vi "Robot Global Data.vi"() -> ()   [LabVIEW 2017]
doc: "This global VI can contain as many global variables as you need. Place a control on the panel, give it a good name. To read or write to it from a VI, drag the icon to the diagram of that VI. You can also drag from the project. Click on the node to change which global you access. You shouldn't have multiple locations writing to a global or it will cause a race-condition."
uses:
  <vilib>/Rock Robotics/WPI/Camera/WPI_CameraImageSize.ctl
  <vilib>/Rock Robotics/WPI/DriverStation/WPI_DriverStationRobotMode2.ctl
  <vilib>/Rock Robotics/WPI/Solenoid/WPI_SolenoidValue.ctl
  <vilib>/Rock Robotics/WPI/DriverStation/WPI_DriverStationMatch Info.ctl
panel:
  in  "Angle at Start of Auto":dbl
  in  "Place From Null":bool
  in  "Auto Selector":string
  in  "Auto Arm Fast":bool
  in  "Lift Down Speed Fast":dbl=-0.9
  in  "Lift Down Fast":bool=TRUE
  in  "Auto Running":dbl=-1.0
  in  "Scale Position":string
  in  "Switch Position":string
  in  "Attempt 2 Cube":bool
  in  "Do Not Cross Field":bool
  in  "Focus Switch":bool
  in  "Have Cube?":bool
  in  "Arm Auto Min Speed":bool
  in  "Cube Sensor":dbl
  in  "Arm Encoder New Reading":dbl
  in  "Auto Scale Drive Forward Distance":dbl=300.0
  in  "Arm Encoder Offset":dbl
  in  "Climbing Override":bool
  in  "Encoders to use":u16(ring)=2 items=["Use Both Encoders", "Use Just Right Encoder", "Use Just Left Encoder"]
  in  "Rollover":dbl
  in  "Continuos Yaw":dbl
  in  "Lift Max Height":dbl=67.0
  out "Match Info":T1={"Autonomous Elapsed Seconds"=0.0, "TeleOp Elapsed Seconds"=0.0, "Disabled Elapsed Seconds"=0.0, "Visited Autonomous"=FALSE, "Visited TeleOp"=FALSE, "Visited Disabled"=FALSE, "Autonomous Settings"={"Autonomous Style"=enum."Independent", "VI Refnum"=refnum}}
  in  "Intake Speed Override":dbl
  in  "Intake Indicator":bool
  in  "Intake Pistons":T2
  in  "Arm Manual Speed":dbl
  in  "Arm Manual Control":bool=TRUE
  in  "LED Control Pattern":dbl=0.27
  in  "LEDs on Robot":bool
  in  "Lift Manual Control":bool
  in  "Lift Manual Speed":dbl
  in  "Intake Speed":dbl
  in  "Right Climber Piston":bool
  in  "Left Climber Piston":bool
  in  "Right Ski Piston":bool
  in  "Left Ski Piston":bool
  in  "Arm Back Limit Switch":bool
  in  "Arm Front Limit Switch":bool
  in  "Lift Encoder Stopped":bool
  in  "Lift Encoder Rate":dbl
  in  "Left Bottom Lift Limit Switch":bool
  in  "Right Bottom Lift Limit Switch":bool
  in  "Left Top Lift Limit Switch":bool
  in  "Right Top Lift Limit Switch":bool
  in  "Lift Encoder Distance":dbl
  in  "Skis on Robot":bool
  in  "Climber on Robot":bool
  in  "Drive on Robot":bool=TRUE
  in  "Intake on Robot":bool=TRUE
  in  "Lift on Robot":bool=TRUE
  in  "Arm on Robot":bool=TRUE
  in  "Practice Bot?":bool
  in  "Compressor Stop":bool
  in  "Lift Height to rase to (in)":dbl
  in  "Lift Max Speed to Raise at (%)":dbl=1.0
  in  "Arm Max Speed to Turn at":dbl
  in  "Arm Angle to Turn to":dbl=3000.0
  in  "Arm Encoder Reading":dbl
  in  "Limelight Pipeline":dbl
  in  "Limelight Cam Mode":dbl=1.0
  in  "Limelight Led Mode":dbl=1.0
  in  "Right Drive Encoder Stopped":bool
  in  "Right Drive Encoder Rate":dbl
  in  "Right Drive Encoder Distance":dbl
  in  "Left Drive Encoder Stopped":bool
  in  "Left Drive Encoder Rate":dbl
  in  "Left Drive Encoder Distance":dbl
  in  "Limelight Data":T3
  in  "Robot Drive Y":dbl
  in  "Robot Drive X":dbl
  in  "Fused Heading":dbl
  in  "Heading":dbl
  in  "Pitch":dbl
  in  "Roll":dbl
  in  "Yaw":dbl
  in  "image size":T4=enum."320x240"
  in  "Enable Vision":bool
  in  "Robot Mode":T5
  # "0 Both\n1 Right\n2 Left"
  # "Navx Data"
  # "Limelight Controls"
  # "Drive Encoders"
  # "Arm"
  # "Items on Robot"
  # "Intake"
  # "Skis"
  # "Climber"
  # "Pnuematics"
  # "Robot Drive Setpoints"
  # "Driver Camera Settings"
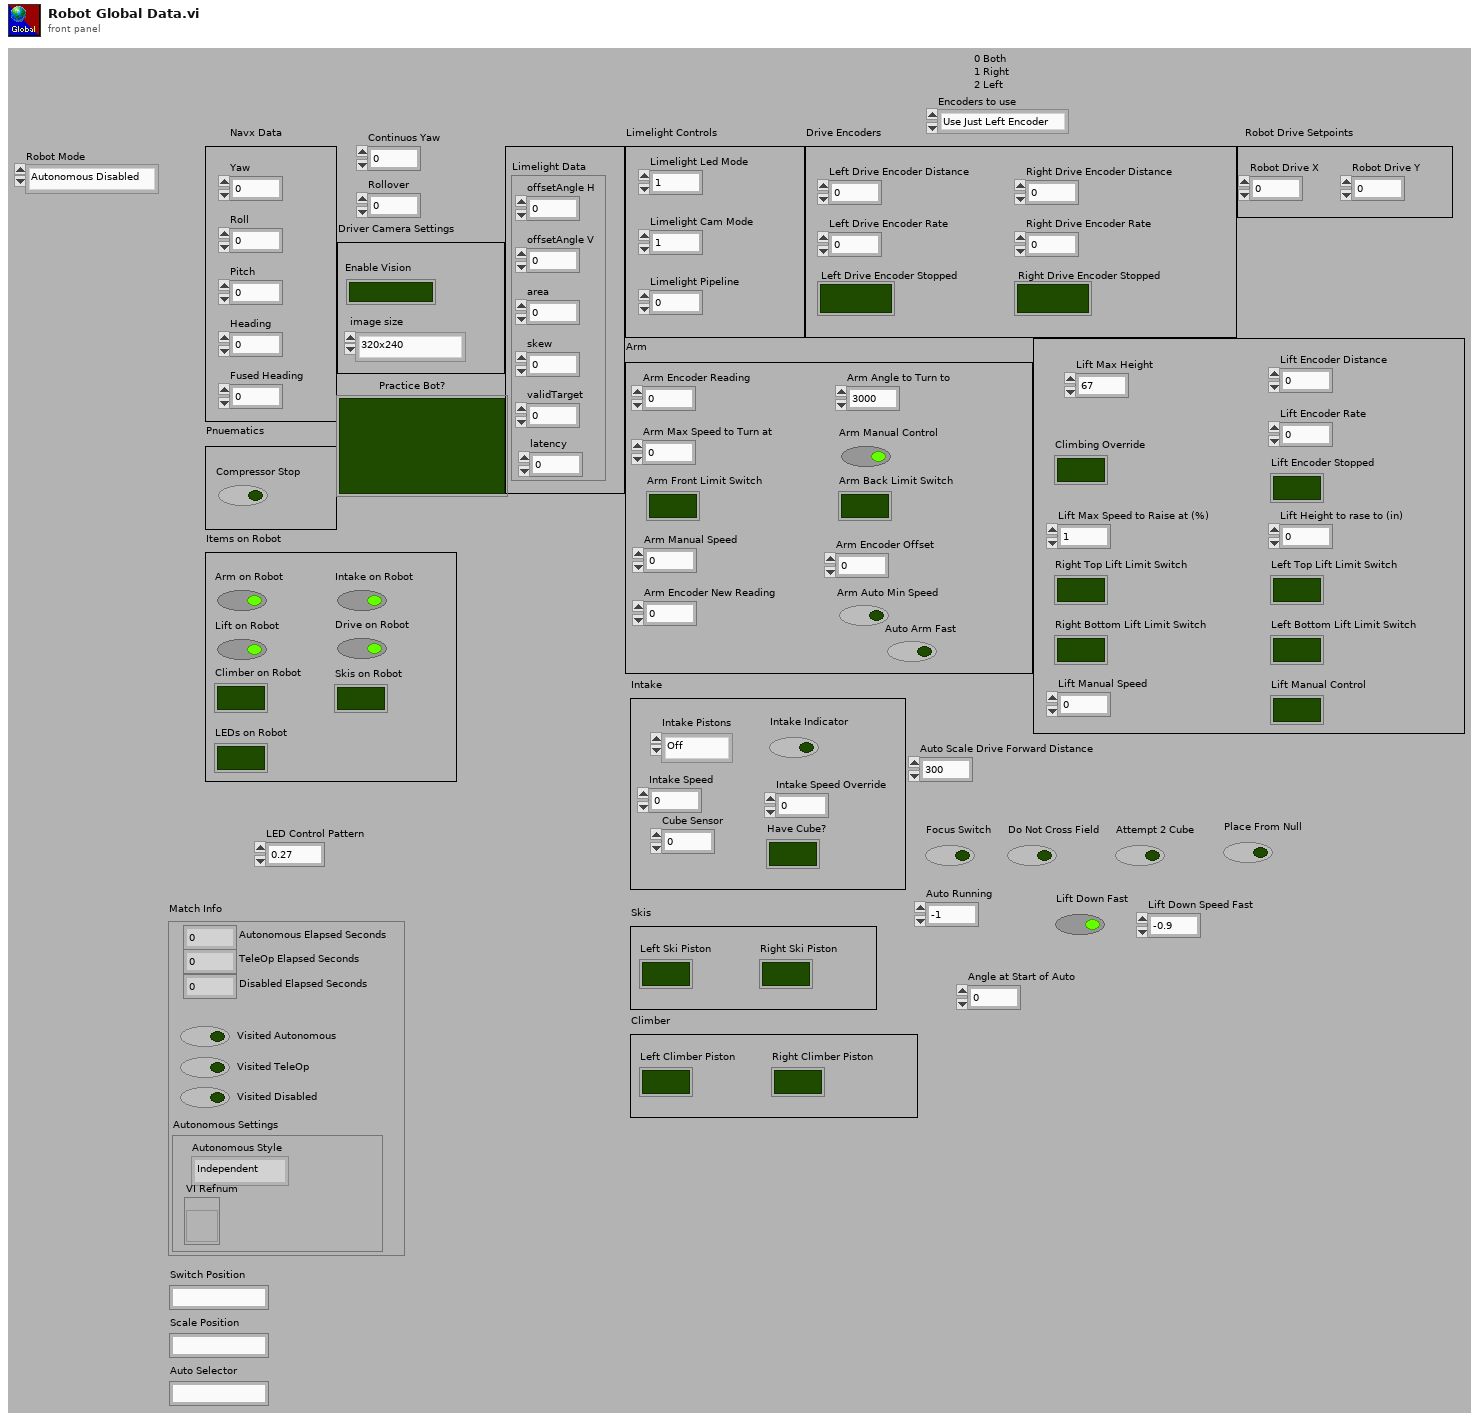
[diagram p1: front panel]
types:
  T1 = typedef "WPI_DriverStationMatch Info.ctl" = cluster{"Autonomous Elapsed Seconds":dbl, "TeleOp Elapsed Seconds":dbl, "Disabled Elapsed Seconds":dbl, "Visited Autonomous":bool, "Visited TeleOp":bool, "Visited Disabled":bool, "Autonomous Settings":cluster{"Autonomous Style":enum16{"Iterative", "Independent"}, "VI Refnum":refnum<vi>}}
  T2 = typedef "WPI_SolenoidValue.ctl" = enum16{"Off", "On", "Forward", "Reverse"}
  T3 = cluster{"offsetAngle H":dbl, "offsetAngle V":dbl, "area":dbl, "skew":dbl, "validTarget":dbl, "latency":dbl}
  T4 = typedef "WPI_CameraImageSize.ctl" = enum16{"640x480", "320x240", "160x120", "Custom"}
  T5 = typedef "WPI_DriverStationRobotMode2.ctl" = enum16{"Autonomous Disabled", "Autonomous Enabled", "Teleop Disabled", "Teleop Enabled", "Disconnected", "Finish", "Test Disabled", "Test Enabled", "Emergency Stopped"}
diagram:
